vi "Table Color Example.vi"() -> ()   [LabVIEW 2016]
uses:
  <vilib>/Utility/miscctls.llb/LVRowAndColumnTypeDef.ctl
panel:
  in  "stop":bool
  in  "Set Color":bool
  in  "Color":u32(colorbox)
  in  "Column":i32
  in  "Row":i32
  in  "Column Headers":string[](array[string])
  in  "Row Headers":string[](array[string])=["RH 1", "RH2 2", "RH 3"]
  out "Table":string[][](table)
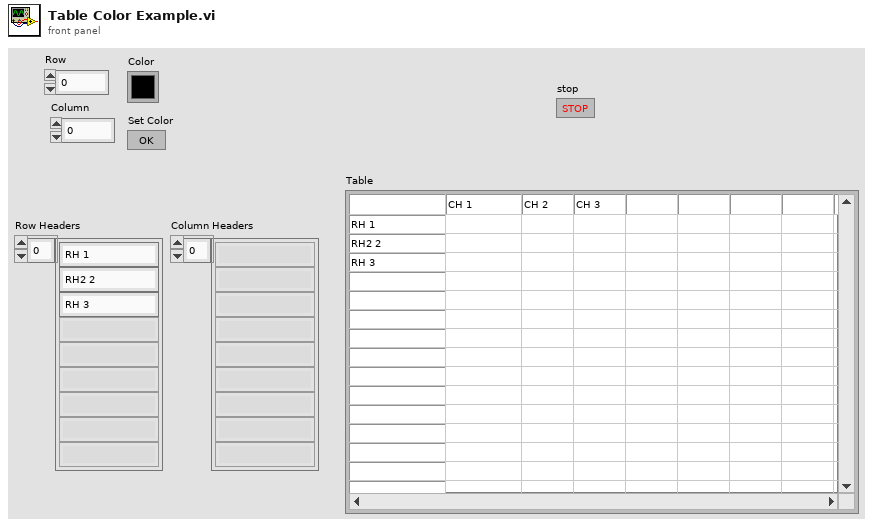
[diagram p1: front panel]
types:
  T1 = typedef "LVRowAndColumnTypeDef.ctl" = cluster{"Row":i32, "Column":i32}
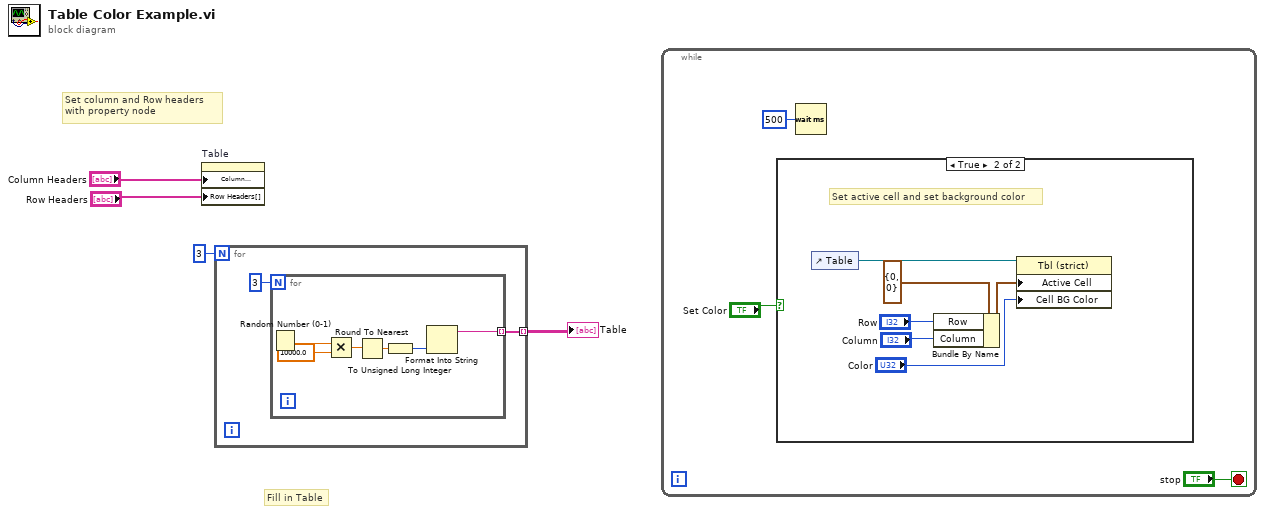
[diagram p0: block diagram]
diagram:
  # "Fill in Table"
  # "Set column and Row headers \nwith property node"
  n1 = property on="Table" class="Tbl (strict)"("Column Headers[]"="Column Headers", "Row Headers[]"="Row Headers") -> ()  [unwired: 2 in, 2 out]
  n2 = for {
    N: 3 -> [_]
    tunnel: [w5] -> w3 mode=indexing
    n3 = for {
      N: 3 -> [_]
      tunnel: [w7] -> w5 mode=indexing
      n4 = Random Number (0-1)() -> (number: 0 to 1=w12:dbl)
      n5 = Multiply(x=w12, y=10000.0) -> (x*y=w10:dbl)
      n6 = Round To Nearest(number=w10) -> (nearest integer value=w9:dbl)
      n7 = To Unsigned Long Integer(number=w9) -> (unsigned 32bit integer=w8:u32)
      n8 = Format Into String(w8) -> (resulting string=w7:string)  [unwired: 3 in, 1 out]
    }
  }
  "Table" <- w3
  n9 = while {
    stop <- "stop" stop-if-true
    n10 = case shown="True" "Set Color" {
      frame False {
      }
      frame True {
        # "Set active cell and set background color"
        n11 = control-ref of="Table"() -> (w21:refnum<vi>)
        n12 = Bundle By Name(cluster=T1 {"Row"=0, "Column"=0} ("Active Cell:Active Cell"), "Row"="Row", "Column"="Column") -> (w19:T1)
        n13 = property class="Tbl (strict)"(reference=w21, "Active Cell"=w19, "Cell BG Color"="Color") -> ()  [unwired: 1 in, 2 out]
      }
    }
    n14 = Wait (ms)(milliseconds to wait=u32 500) -> ()  [unwired: 1 out]
  }
